vi "ISM Reserve Pump.vi"(8 "error in (no error)":errorcluster, 10 "ISM Channel # In":i32, 11 "ISM Pump # In":i32) -> (0 "error out":errorcluster, 2 "Loop Completed":bool, 3 "ISM Pump # Out":i32)   [LabVIEW 2018, in "Ismatec 4308.lvlib"]
uses:
  Ismatec 4308.lvlib
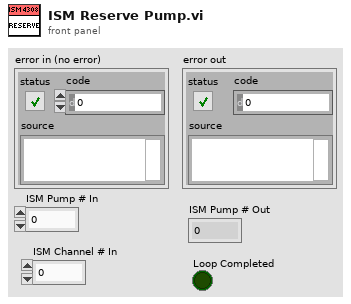
[diagram p1: front panel]
types:
  T1 = cluster{"Busy":bool, "ChannelCnt":dbl, "Initialized":bool, "Current Channel":dbl, "Initialized Channels":dbl[]}[]
  T2 = cluster{"Busy":bool, "ChannelCnt":dbl, "Initialized":bool, "Current Channel":dbl, "Initialized Channels":dbl[]}
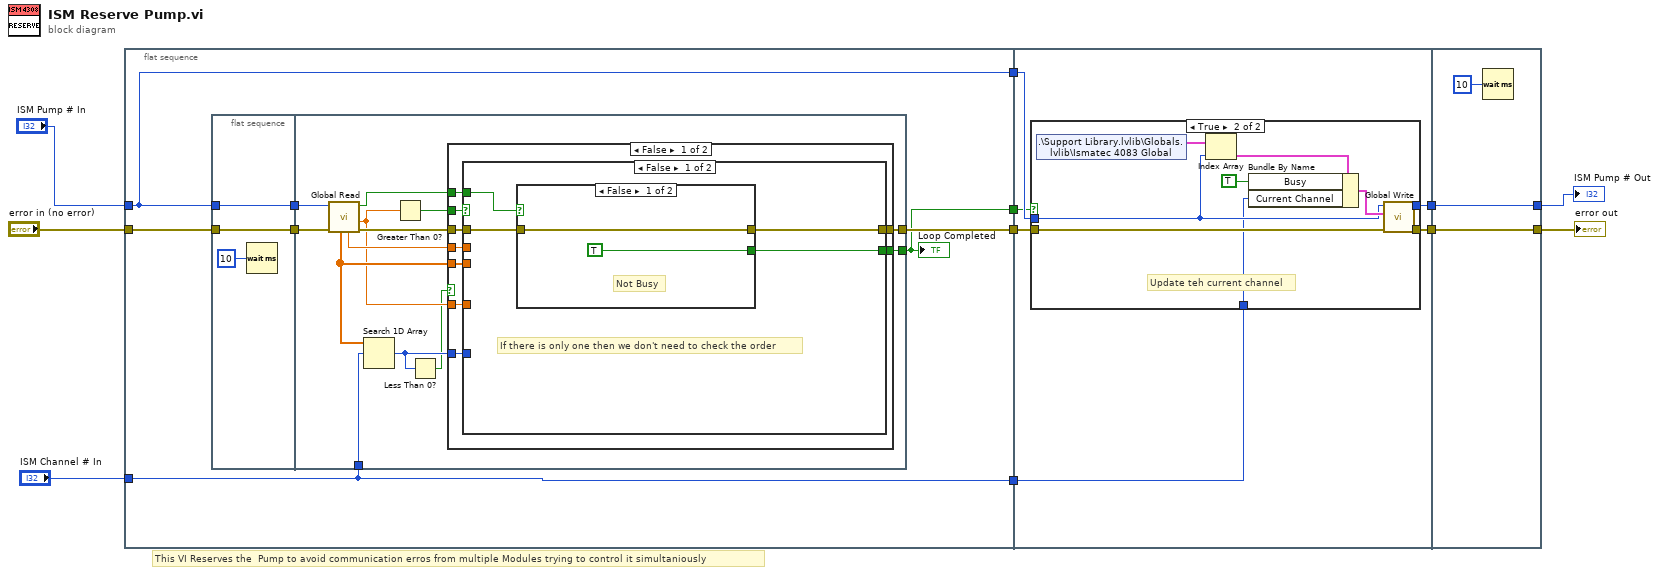
[diagram p0: block diagram]
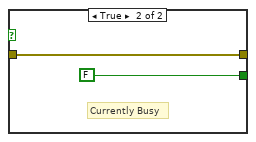
[diagram p2: hidden frame]
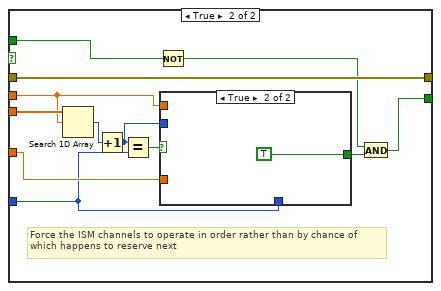
[diagram p3: hidden frame]
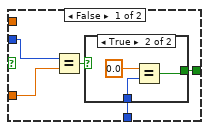
[diagram p4: hidden frame]
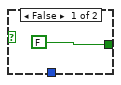
[diagram p5: hidden frame]
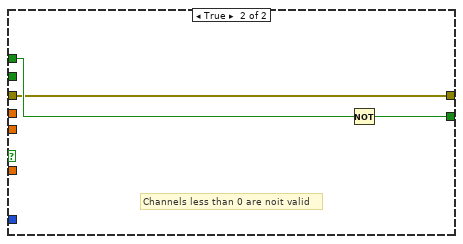
[diagram p6: hidden frame]
diagram:
  # "This VI Reserves the  Pump to avoid communication erros from multiple Modules trying to control it simultaniously"
  n1 = flat-sequence {
    tunnel: [w17] -> w9
    tunnel: [w16] -> w8
    tunnel: "error in (no error)" -> [w18]
    tunnel: [w15] -> w6
    tunnel: "ISM Pump # In" -> [w16]
    tunnel: "ISM Channel # In" -> [w15]
    tunnel: [w12] -> w1
    tunnel: [w81] -> w11
    tunnel: w9 -> [w82]
    tunnel: w8 -> [w80]
    tunnel: w6 -> [w79]
    tunnel: [w78] -> w2
    tunnel: w1 -> [w77]
    tunnel: [w96] -> w10
    tunnel: w11 -> [w96]
    tunnel: [w94] -> w3
    tunnel: w2 -> [w94]
    frame #0 {
      n2 = flat-sequence {
        tunnel: [w21] -> w14
        tunnel: w18 -> [w21]
        tunnel: w16 -> [w20]
        tunnel: [w20] -> w13
        tunnel: [w28] -> w17
        tunnel: [w30] -> w12
        tunnel: w14 -> [w34]
        tunnel: w13 -> [w33]
        tunnel: w15 -> [w24]
        frame #0 {
          n3 = Wait (ms)(milliseconds to wait=u32 10) -> ()  [unwired: 1 out]
        }
        frame #1 {
          n4 = call "Global Read.vi"("error in (no error)"=w34, "Pump Number"=w33) -> ("error out"=w29:errorcluster, "ChannelCnt"=w25:dbl, "Busy"=w31:bool, "Current Channel"=w27:dbl, "Initialized Channels"=w26:dbl[])  [unwired: 3 in, 2 out]
          n5 = Search 1D Array(1D array=w26, element=w24) -> (index of element=w23:i32)  [unwired: 1 in]
          n6 = Greater Than 0?(x=w25) -> (x > 0?=w32:bool)
          n7 = Less Than 0?(x=w23) -> (x < 0?=w22:bool)
          n8 = case shown="False" w22 {
            tunnel: w32 -> [w43 _]
            tunnel: w31 -> [w42 w76]
            tunnel: [w41 w75] -> w30
            tunnel: w29 -> [w40 w74]
            tunnel: [w39 w74] -> w28
            tunnel: w27 -> [w38 _]
            tunnel: w26 -> [w37 _]
            tunnel: w25 -> [w36 _]
            tunnel: w23 -> [w35 _]
            frame False {
              n9 = case shown="False" w43 {
                tunnel: w42 -> [w47 w61]
                tunnel: [w46 w60] -> w41
                tunnel: w40 -> [w45 w62]
                tunnel: [w44 w62] -> w39
                tunnel: w37 -> [_ w63]
                tunnel: w38 -> [_ w55]
                tunnel: w36 -> [_ w56]
                tunnel: w35 -> [_ w53]
                frame False {
                  # "If there is only one then we don't need to check the order"
                  n10 = case shown="False" w47 {
                    tunnel: [TRUE FALSE] -> w46
                    tunnel: w45 -> [w48 w50]
                    tunnel: [w48 w50] -> w44
                    frame False {
                      # "Not Busy"
                    }
                    frame True {
                      # "Currently Busy"
                    }
                  }
                }
                frame True {
                  # "Force the ISM channels to operate in order rather than by chance of\nwhich happens to reserve next"
                  n11 = Search 1D Array(1D array=w63, element=w55) -> (index of element=w54:i32)  [unwired: 1 in]
                  n12 = Increment(x=w54) -> (x+1=w52:i32)
                  n13 = Equal?(x=w52, y=w53) -> (x = y?=w59:bool)
                  n14 = Not(x=w61) -> (.not. x?=w58:bool)
                  n15 = case shown="True" w59 {
                    tunnel: [w68 TRUE] -> w57
                    tunnel: w56 -> [w67 _]
                    tunnel: w55 -> [_ _]
                    tunnel: w53 -> [w65 _]
                    tunnel: w52 -> [w64 _]
                    frame False {
                      n16 = Equal?(x=w64, y=w67) -> (x = y?=w66:bool)
                      n17 = case shown="True" w66 {
                        tunnel: [FALSE w70] -> w68
                        tunnel: w65 -> [_ w71]
                        frame False {
                        }
                        frame True {
                          n18 = Equal?(x=0.0, y=w71) -> (x = y?=w70:bool)
                        }
                      }
                    }
                    frame True {
                    }
                  }
                  n19 = And(x=w58, y=w57) -> (x .and. y?=w60:bool)
                }
              }
            }
            frame True {
              # "Channels less than 0 are noit valid"
              n20 = Not(x=w76) -> (.not. x?=w75:bool)
            }
          }
        }
      }
      "Loop Completed" <- w12
    }
    frame #1 {
      n21 = case shown="True" w77 {
        tunnel: w82 -> [w84 w93]
        tunnel: [w84 w92] -> w81
        tunnel: w80 -> [w83 w87]
        tunnel: w79 -> [_ w86]
        tunnel: [w83 w85] -> w78
        frame False {
        }
        frame True {
          # "Update teh current channel"
          n22 = shared-variable ".\\Support Library.lvlib\\Globals.lvlib\\Ismatec 4083 Global"() -> (w91:T1)  [unwired: 1 in, 1 out]
          n23 = Index Array(array=w91, index=w87) -> (element=w88:T2)
          n24 = Bundle By Name(cluster=w88, "Busy"=TRUE, "Current Channel"=w86) -> (w89:T2)
          n25 = call "Global Write.vi"("error in (no error)"=w93, "Incoming Cluster"=w89, "Pump Number In"=w87) -> ("error out"=w92:errorcluster, "Pump Number Out"=w85:i32)  [unwired: 7 in]
        }
      }
    }
    frame #2 {
      n26 = Wait (ms)(milliseconds to wait=u32 10) -> ()  [unwired: 1 out]
    }
  }
  "error out" <- w10
  "ISM Pump # Out" <- w3
